vi "Update SubPanel Size.vi"(8 "错误输入（无错误）":errorcluster, 10 "窗口边界":T1, 11 "SubPanel输入":refnum<vi>) -> (0 "错误输出":errorcluster)   [LabVIEW 2018, in "MainInterface.lvlib"]
uses:
  MainInterface.lvlib
  <vilib>/Utility/miscctls.llb/LVRectTypeDef.ctl
  <vilib>/Utility/miscctls.llb/LVBoundsTypeDef.ctl
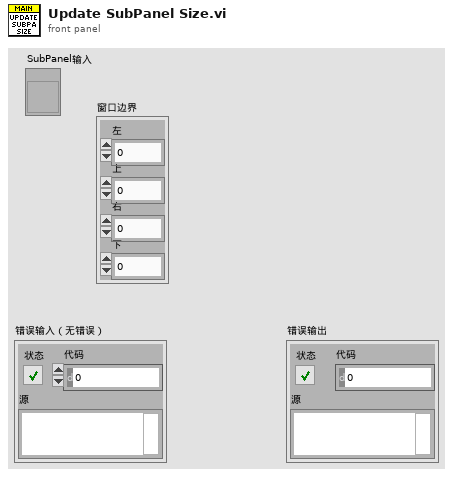
[diagram p1: front panel]
types:
  T1 = typedef "LVRectTypeDef.ctl" = cluster{"Left":i16, "Top":i16, "Right":i16, "Bottom":i16}
  T2 = typedef "LVBoundsTypeDef.ctl" = cluster{"Width":u32, "Height":u32}
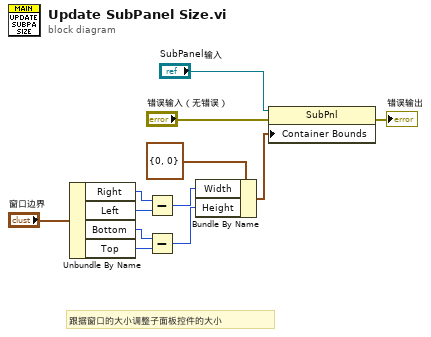
[diagram p0: block diagram]
diagram:
  # "跟据窗口的大小调整子面板控件的大小"
  n1 = Unbundle By Name("窗口边界") -> ("Right"=w7:i16, "Left"=w8:i16, "Bottom"=w10:i16, "Top"=w11:i16)
  n2 = Subtract(x=w7, y=w8) -> (x-y=w9:i16)
  n3 = Subtract(x=w10, y=w11) -> (x-y=w12:i16)
  n4 = Bundle By Name(cluster=T2 {"Width"=0, "Height"=0} ("容器边界"), "Width"=w9, "Height"=w12) -> (w5:T2)
  n5 = property class="SubPnl"(reference="SubPanel输入", error in="错误输入（无错误）", "Container Bounds"=w5) -> (error out=→"错误输出":errorcluster)  [unwired: 1 out]
